vi "Write Unique Identifier 2.vi"(8 "error in (no error)":errorcluster, 10 "Unique Identifier":string, 11 "Function in":refnum<class "Function.lvclass">) -> (0 "error out":errorcluster, 3 "Function out":refnum<class "Function.lvclass">)   [LabVIEW 2016, in "Function Actor.lvlib" / "Function.lvclass"]
uses:
  <userlib>/Common Components/Function Actor/Function.lvclass
  <userlib>/Common Components/Function Actor/Function.lvclass/Function.ctl
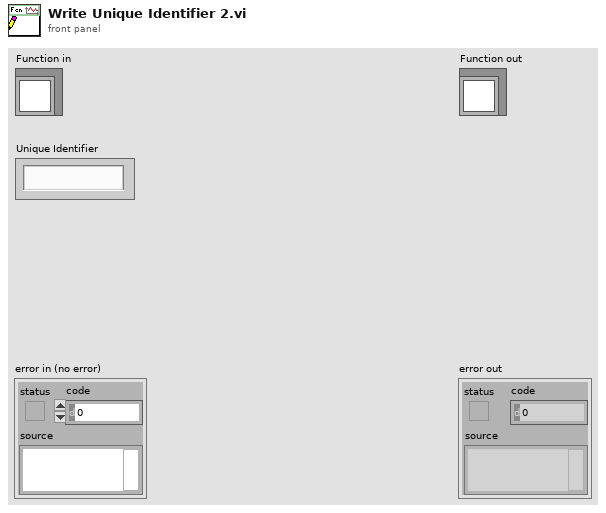
[diagram p1: front panel]
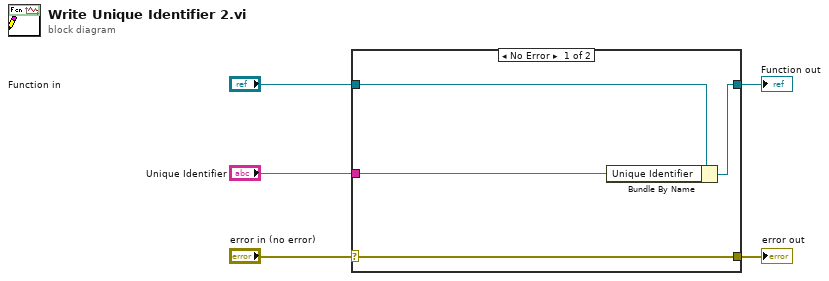
[diagram p0: block diagram]
diagram:
  n1 = case shown="No Error" "error in (no error)" {
    selector: "error in (no error)" -> [w9 w10]
    tunnel: [w9 w10] -> w4
    tunnel: [w7 w11] -> w2
    tunnel: "Function in" -> [w8 w11]
    tunnel: "Unique Identifier" -> [w6 _]
    frame No Error {
      n2 = Bundle By Name(cluster=w8, "Unique Identifier"=w6) -> (w7:refnum<class "Function.lvclass">)
    }
    frame Error {
    }
  }
  "error out" <- w4
  "Function out" <- w2
